vi "LaptopClient2modes.vi"() -> ()   [LabVIEW 2018]
uses:
  Modes.ctl
  <vilib>/daq.io/MQTT LabVIEW Client/Controls/QoS.ctl
  <vilib>/daq.io/MQTT LabVIEW Client/Controls/DUP_Flag.ctl
  <vilib>/daq.io/MQTT LabVIEW Client/Controls/Retain_Flag.ctl
  <vilib>/daq.io/MQTT LabVIEW Client/Controls/Connect_Flags.ctl
  <vilib>/daq.io/MQTT LabVIEW Client/MQTT_Functions.lvlib
panel:
  in  "Bulb":bool
  in  "Fan":bool
  in  "Mode Control":bool
  out "Mode":T1
  in  "stop":bool
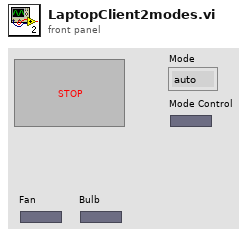
[diagram p1: front panel]
types:
  T1 = typedef "Modes.ctl" = enum16{"auto", "manual"}
  T2 = typedef "MQTT_Functions.lvlib/QoS.ctl" = enum8{"At most once", "At least once", "Exactly once", "Reserved"}
  T3 = typedef "MQTT_Functions.lvlib/Connect_Flags.ctl" = cluster{"user name":bool, "password":bool, "will retain":bool, "will flag":bool, "clean session":bool, "reserved":bool, "will QoS":T2}
  T4 = typedef "MQTT_Functions.lvlib/DUP_Flag.ctl" = bool
  T5 = typedef "MQTT_Functions.lvlib/Retain_Flag.ctl" = bool
  T6 = cluster{"QoS":T2, "DUP":T4, "Retain":T5, "Keep Alive (sec)":u16}
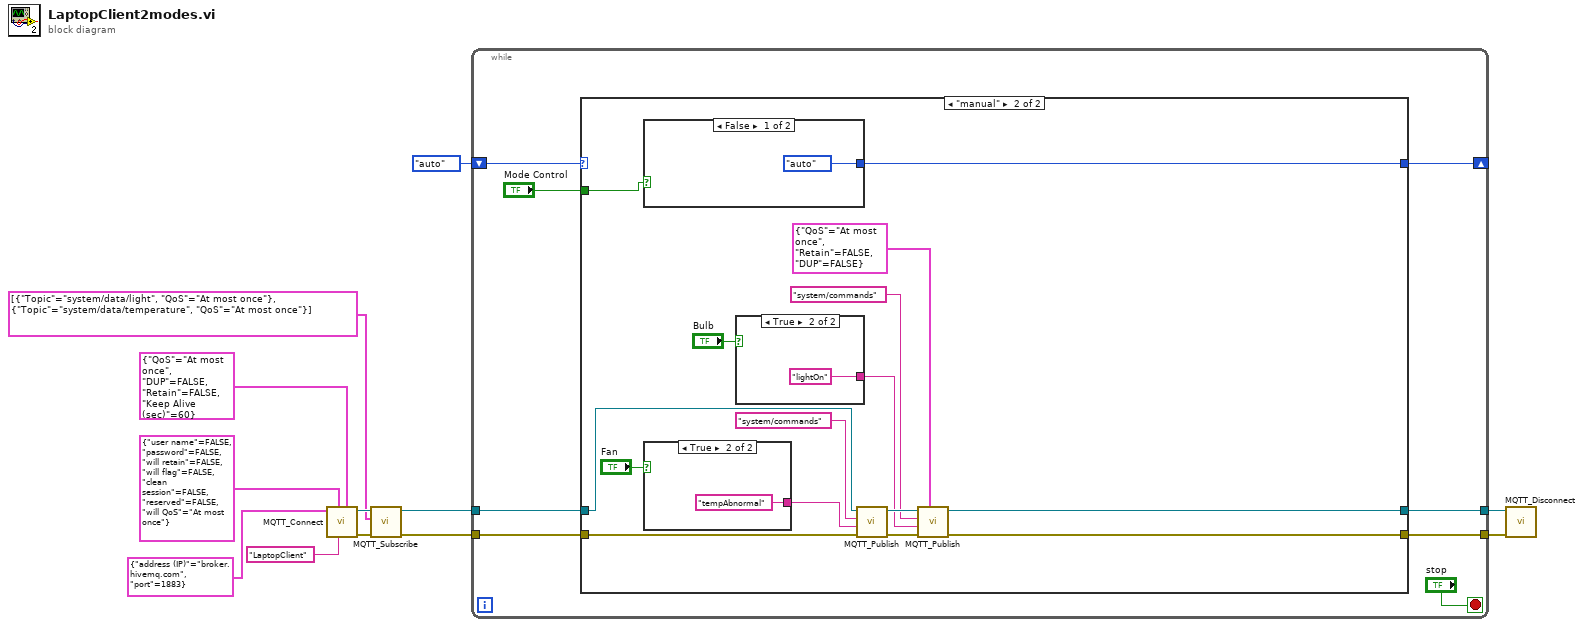
[diagram p0: block diagram]
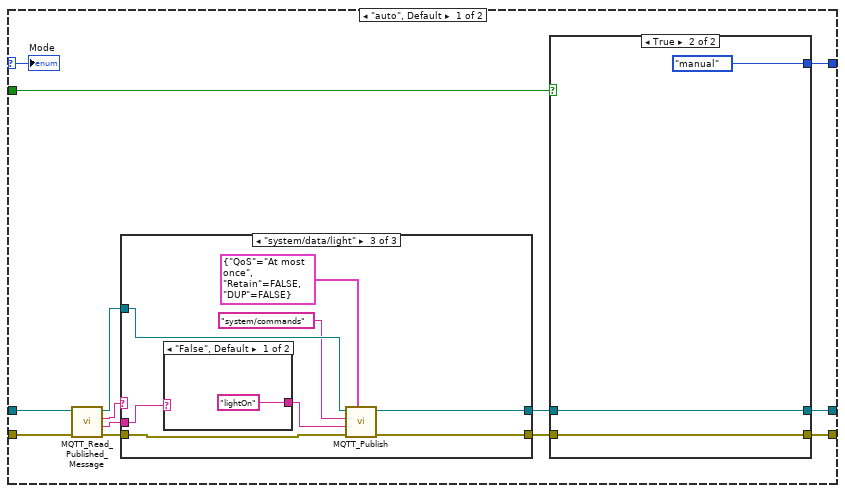
[diagram p2: hidden frame]
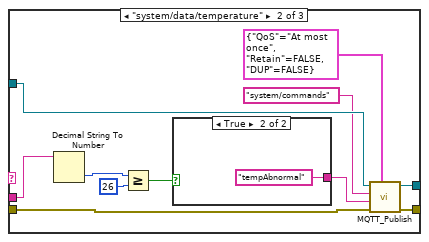
[diagram p4: hidden frame]
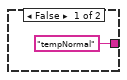
[diagram p5: hidden frame]
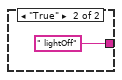
[diagram p6: hidden frame]
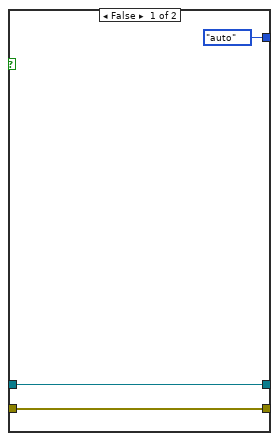
[diagram p7: hidden frame]
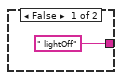
[diagram p8: hidden frame]
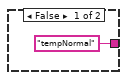
[diagram p9: hidden frame]
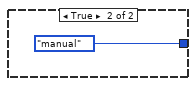
[diagram p10: hidden frame]
diagram:
  n1 = call <vilib>:"MQTT_Connect.vi"("Connect Meta"=T6 {"QoS"=enum."At most once", "DUP"=FALSE, "Retain"=FALSE, "Keep Alive (sec)"=60}, "Client ID"="LaptopClient", "Connect Flags"=T3 {"user name"=FALSE, "password"=FALSE, "will retain"=FALSE, "will flag"=FALSE, "clean session"=FALSE, "reserved"=FALSE, "will QoS"=enum."At most once"}, "MQTT Broker"=cluster{"address (IP)":string, "port":u16} {"address (IP)"="broker.hivemq.com", "port"=1883}) -> ("error out"=w6:errorcluster, "connection ID out"=w7:refnum<k5>)  [unwired: 5 in, 1 out]
  n2 = call <vilib>:"MQTT_Subscribe.vi"("error in (no error)"=w6, "Subscription Info Array"=cluster{"Topic":string, "QoS":T2}[] [{"Topic"="system/data/light", "QoS"=enum."At most once"}, {"Topic"="system/data/temperature", "QoS"=enum."At most once"}], "connection ID"=w7) -> ("error out"=w4:errorcluster, "connection ID out"=w3:refnum<k5>)  [unwired: 7 in]
  n3 = while {
    shift-right: [w18] -> _
    shift-left: Modes."auto" -> [w20]
    tunnel: w4 -> [w16]
    tunnel: w3 -> [w15]
    tunnel: [w14] -> w1
    tunnel: [w13] -> w2
    stop <- "stop" stop-if-true
    n4 = case shown="\"manual\"" w20 {
      selector: w20 -> [w33 _]
      tunnel: [w32 w78] -> w18
      tunnel: "Mode Control" -> [w31 w79]
      tunnel: w16 -> [w30 w74]
      tunnel: w15 -> [w29 w75]
      tunnel: [w22 w66] -> w14
      tunnel: [w21 w65] -> w13
      frame "auto", Default {
        n5 = call <vilib>:"MQTT_Read_Published_Message.vi"("error in (no error)"=w30, "connection ID"=w29) -> ("error out"=w26:errorcluster, "Message"=w27:string, "Topic Name"=w28:string, "connection ID out"=w24:refnum<k5>)  [unwired: 4 in, 2 out]
        n6 = case shown="\"system/data/light\"" w28 {
          tunnel: w27 -> [_ w46 w56]
          tunnel: w26 -> [w35 w42 w55]
          tunnel: [w35 w41 w49] -> w25
          tunnel: w24 -> [w34 w38 w53]
          tunnel: [w34 w39 w52] -> w23
          frame "False", Default {
          }
          frame "system/data/temperature" {
            n7 = Decimal String To Number(string=w46) -> (number=w45:i32)  [unwired: 2 in, 1 out]
            n8 = Greater Or Equal?(x=w45, y=26) -> (x >= y?=w43:bool)
            n9 = case shown="True" w43 {
              tunnel: ["tempNormal" ("Message to be published") "tempAbnormal" ("Message to be published")] -> w40
              frame False {
              }
              frame True {
              }
            }
            n10 = call <vilib>:"MQTT_Publish.vi"("Publish Meta"=cluster{"QoS":T2, "Retain":T5, "DUP":T4} {"QoS"=enum."At most once", "Retain"=FALSE, "DUP"=FALSE}, "error in (no error)"=w42, "Message to be published"=w40, "Topic"="system/commands", "connection ID"=w38) -> ("error out"=w41:errorcluster, "connection ID out"=w39:refnum<k5>)  [unwired: 5 in]
          }
          frame "system/data/light" {
            n11 = case shown="\"False\", Default" w56 {
              tunnel: ["lightOn" ("Message to be published") " lightOff" ("Message to be published")] -> w54
              frame "False", Default {
              }
              frame "True" {
              }
            }
            n12 = call <vilib>:"MQTT_Publish.vi"("Publish Meta"=cluster{"QoS":T2, "Retain":T5, "DUP":T4} {"QoS"=enum."At most once", "Retain"=FALSE, "DUP"=FALSE}, "error in (no error)"=w55, "Message to be published"=w54, "Topic"="system/commands", "connection ID"=w53) -> ("error out"=w49:errorcluster, "connection ID out"=w52:refnum<k5>)  [unwired: 5 in]
          }
        }
        n13 = case shown="True" w31 {
          tunnel: [Modes."auto" ("Enum") Modes."manual" ("Enum")] -> w32
          tunnel: w25 -> [w59 w62]
          tunnel: w23 -> [w60 w63]
          tunnel: [w60 w63] -> w22
          tunnel: [w59 w62] -> w21
          frame False {
          }
          frame True {
          }
        }
        "Mode" <- w33
      }
      frame "manual" {
        n14 = case shown="False" w79 {
          tunnel: [Modes."auto" ("Enum") Modes."manual" ("Enum")] -> w78
          frame False {
          }
          frame True {
          }
        }
        n15 = case shown="True" "Fan" {
          tunnel: ["tempNormal" ("Message to be published") "tempAbnormal" ("Message to be published")] -> w73
          frame False {
          }
          frame True {
          }
        }
        n16 = case shown="True" "Bulb" {
          tunnel: [" lightOff" ("Message to be published") "lightOn" ("Message to be published")] -> w69
          frame False {
          }
          frame True {
          }
        }
        n17 = call <vilib>:"MQTT_Publish.vi"("error in (no error)"=w74, "Message to be published"=w73, "Topic"="system/commands", "connection ID"=w75) -> ("error out"=w70:errorcluster, "connection ID out"=w71:refnum<k5>)  [unwired: 6 in]
        n18 = call <vilib>:"MQTT_Publish.vi"("Publish Meta"=cluster{"QoS":T2, "Retain":T5, "DUP":T4} {"QoS"=enum."At most once", "Retain"=FALSE, "DUP"=FALSE}, "error in (no error)"=w70, "Message to be published"=w69, "Topic"="system/commands", "connection ID"=w71) -> ("error out"=w65:errorcluster, "connection ID out"=w66:refnum<k5>)  [unwired: 5 in]
      }
    }
  }
  n19 = call <vilib>:"MQTT_Disconnect.vi"("error in (no error)"=w2, "connection ID"=w1) -> ()  [unwired: 9 in, 1 out]
